vi "Handle Error SM.vi"(7 "NoContinue (F)":bool, 8 "error in (no error)":errorcluster, 10 "CustomMessage":string) -> (0 "error out":errorcluster, 1 "error out Upstream":errorcluster, 2 "Shutdown?":bool)   [LabVIEW 2019, in "ErrorHandler.lvclass"]
doc: "Developed by Kevin Thompson\nkevin@thompsonengineering.net\n\nCopyright 2018\nThompson Engineering, LLC"
uses:
  ErrorHandler.lvclass
  TypeDef/HandleErrorSM - AppData--clustesr.ctl
  <vilib>/Utility/error.llb/DialogType.ctl
  TypeDef/ErrorRemote EventData.ctl
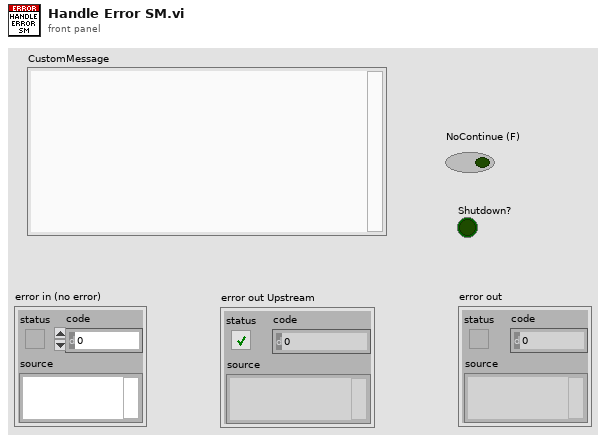
[diagram p1: front panel]
types:
  T1 = typedef "ErrorHandler.lvclass/HandleErrorSM - AppData--clustesr.ctl" = cluster{"error in":errorcluster, "ErrorText":string, "ErrorPathname":path, "ErrorRemoteEventData":T2}
  T2 = typedef "ErrorHandler.lvclass/ErrorRemote EventData.ctl" = cluster{"Timestamp":timestamp, "ErrorCluster":errorcluster, "message":string, "Shutdown?":bool, "DialogDisabled?":bool, "TerminateOnError?":bool}
  T3 = enum16{"Native", "Native Command Line", "UNIX", "Macintosh", "DOS"}
  T4 = typedef "DialogType.ctl" = u16
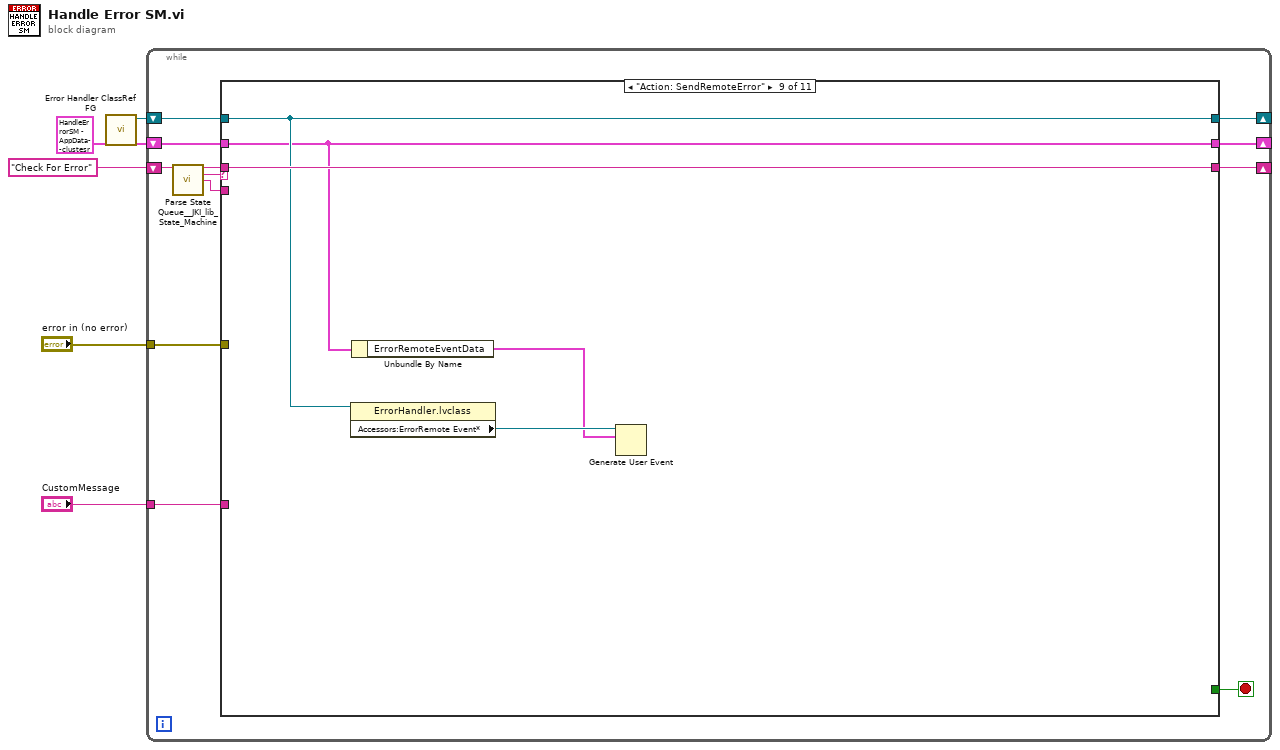
[diagram p0: block diagram]
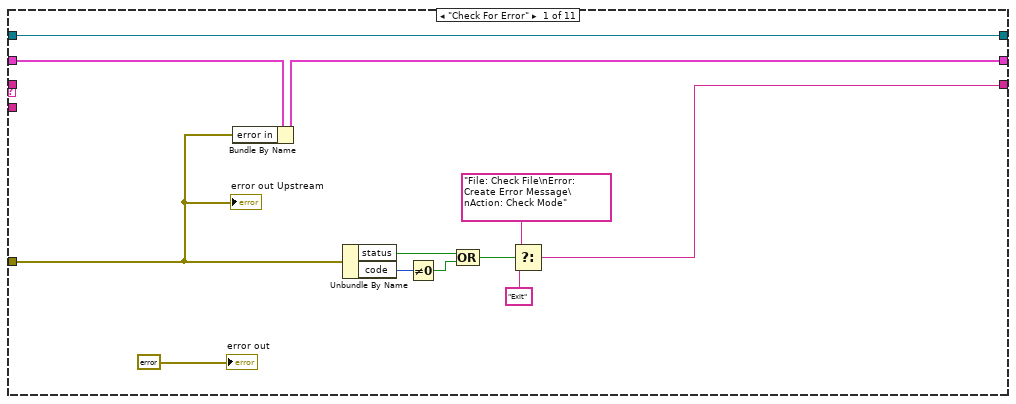
[diagram p2: hidden frame]
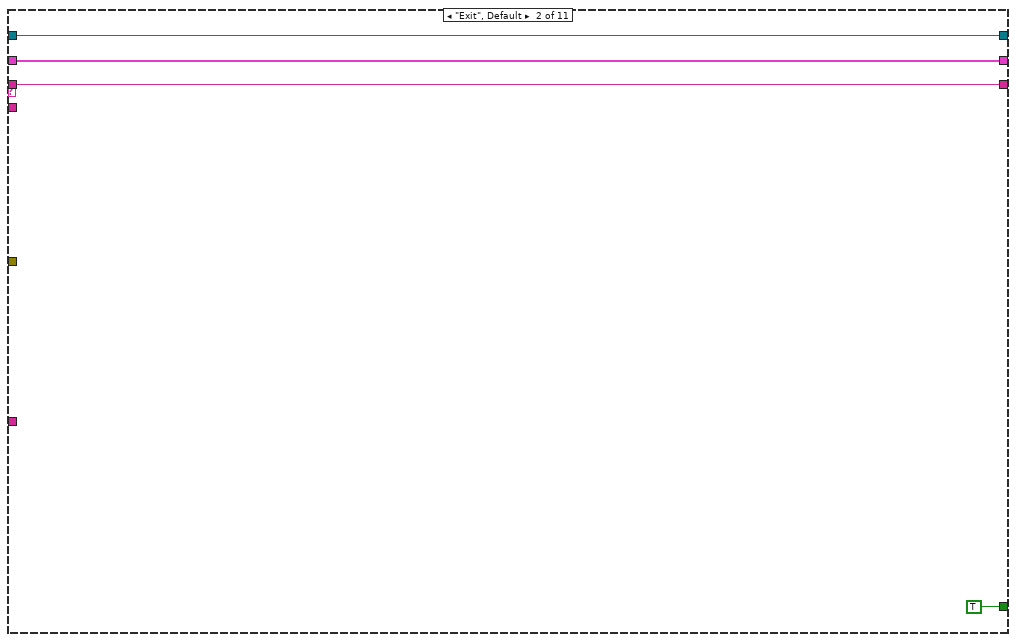
[diagram p3: hidden frame]
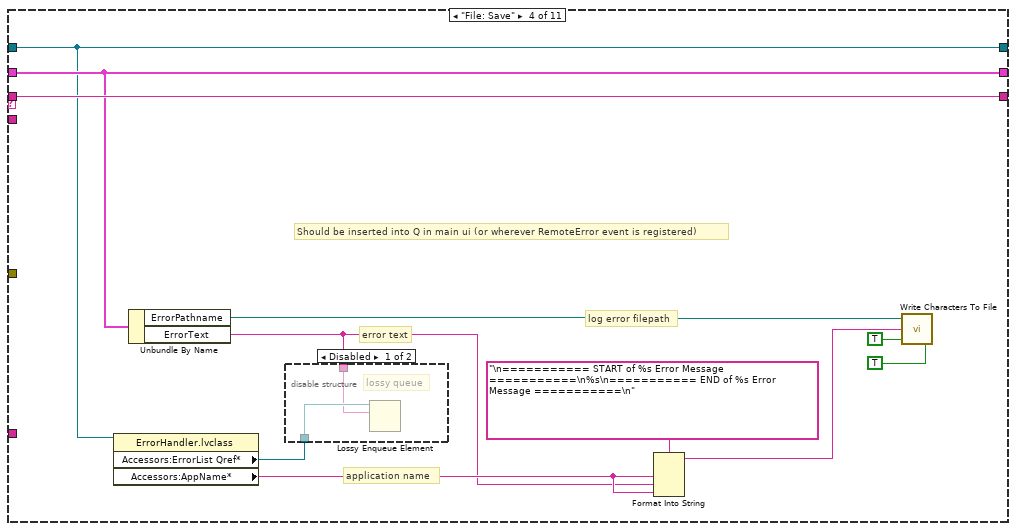
[diagram p5: hidden frame]
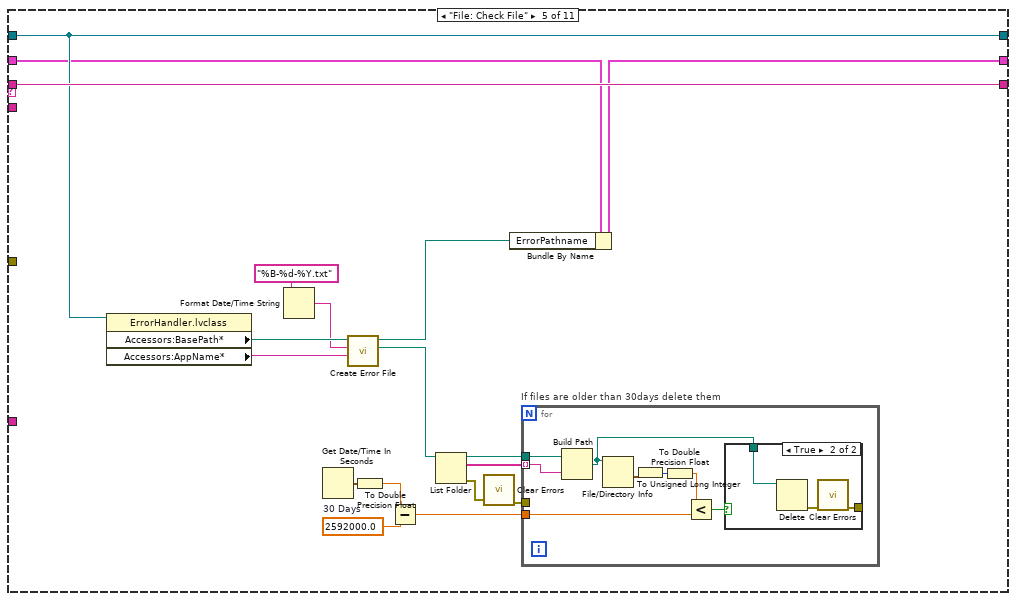
[diagram p7: hidden frame]
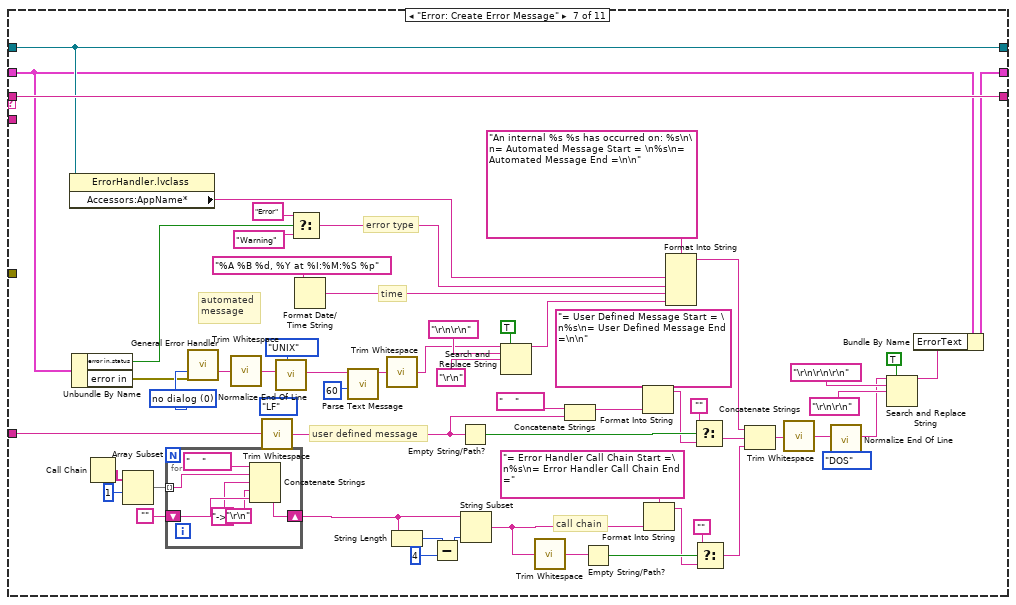
[diagram p10: hidden frame]
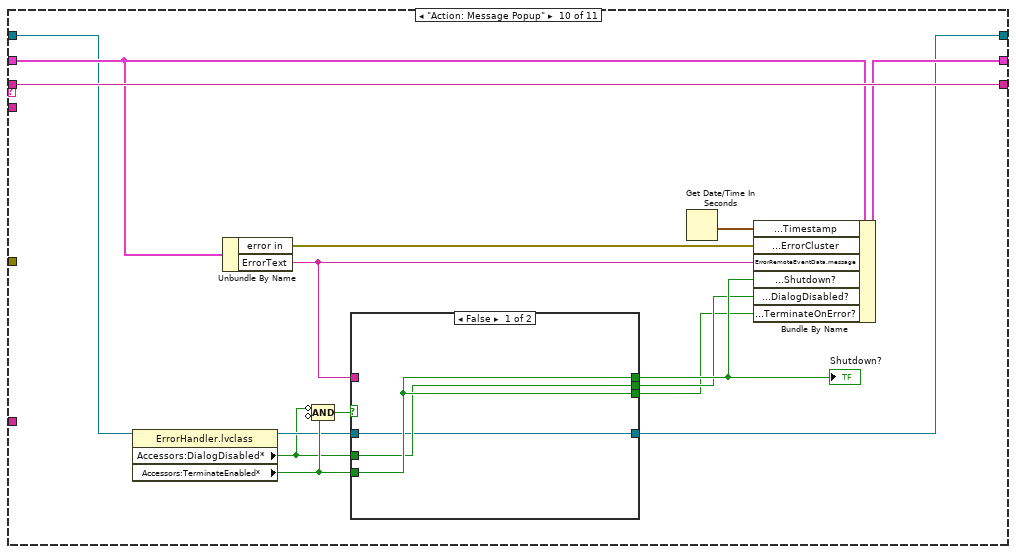
[diagram p12: hidden frame]
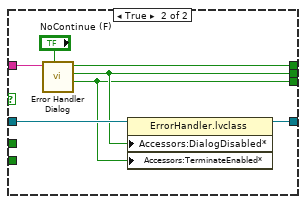
[diagram p13: hidden frame]
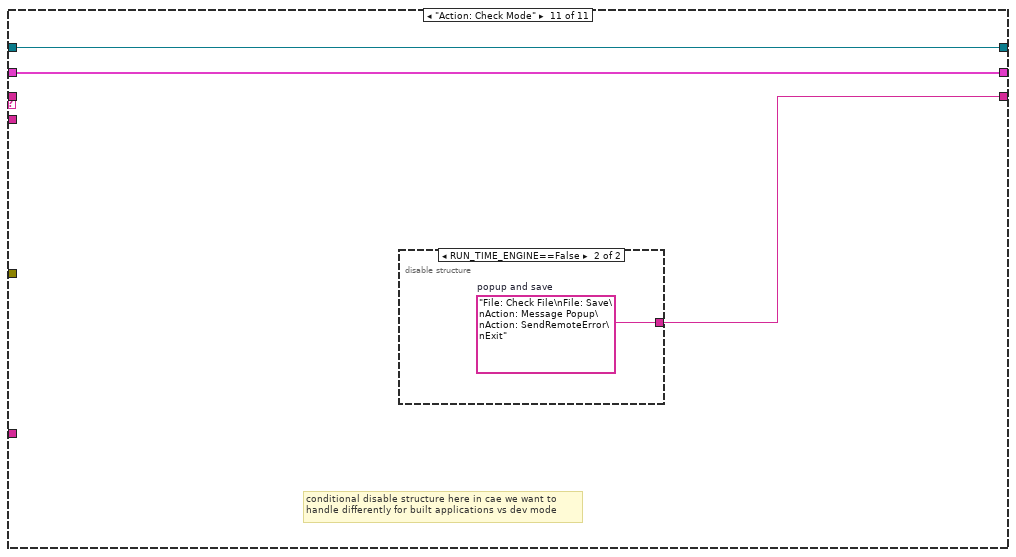
[diagram p14: hidden frame]
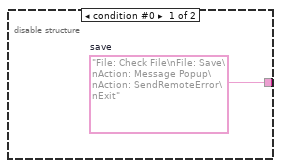
[diagram p15: hidden frame]
diagram:
  n1 = call "Error Handler ClassRef FG.vi"() -> ("ErrorHandler out"=w5:refnum<class "ErrorHandler.lvclass">)  [unwired: 10 in, 1 out]
  n2 = while {
    shift-right: [w14] -> _
    shift-left: "Check For Error" ("Remaining States") -> [w16]
    shift-right: [w11] -> _
    shift-left: w5 -> [w12]
    tunnel: "error in (no error)" -> [w10]
    shift-right: [w8] -> _
    shift-left: T1 {"error in"={"status"=FALSE, "code"=0, "source"=""}, "ErrorText"="", "ErrorPathname"=path "", "ErrorRemoteEventData"={"Timestamp"=timestamp(0 s since 1904-01-01), "ErrorCluster"={"status"=FALSE, "code"=0, "source"=""}, "message"="", "Shutdown?"=FALSE, "DialogDisabled?"=FALSE, "TerminateOnError?"=FALSE}} ("HandleErrorSM AppData") -> [w9]
    tunnel: "CustomMessage" -> [w6]
    stop <- w7 stop-if-true
    n3 = call <vilib>:"Parse State Queue__JKI_lib_State_Machine.vi"("State Queue"=w16) -> ("Remaining States"=w15:string, "Current State"=w17:string, "Arguments"=w13:string)  [unwired: 12 in]
    n4 = case shown="\"Action: SendRemoteError\"" w17 {
      tunnel: w15 -> [_ w33 w36 w47 w67 w81 w139 w148 w153 w168 _]
      tunnel: [w22 w33 w36 w47 w67 w81 w139 w148 w153 w168 w179] -> w14
      tunnel: w13 -> [_ _ _ _ _ _ _ _ _ _ _]
      tunnel: w12 -> [w29 w32 w35 w40 w66 w80 w91 w147 w152 w155 w181]
      tunnel: [w29 w32 w35 w40 w66 w80 w91 w147 w152 w154 w181] -> w11
      tunnel: w10 -> [w19 _ _ _ _ _ _ _ _ _ _]
      tunnel: [w20 w31 w34 w41 w51 w79 w87 w146 w150 w162 w180] -> w8
      tunnel: w9 -> [w21 w31 w34 w41 w52 w79 w88 w146 w150 w163 w180]
      tunnel: [_ TRUE _ _ _ _ _ _ _ _ _] -> w7
      tunnel: w6 -> [_ _ _ _ _ _ w89 _ _ _ _]
      frame "Check For Error" {
        n5 = Bundle By Name(cluster=w21, "error in"=w19) -> (w20:T1)
        n6 = Unbundle By Name(w19) -> ("status"=w28:bool, "code"=w27:i32)
        n7 = Not Equal To 0?(x=w27) -> (x != 0?=w26:bool)
        n8 = Compound Arithmetic op=OR(w28, w26) -> (w25:bool)
        n9 = Select(t="File: Check File\nError: Create Error Message\nAction: Check Mode", s=w25, f="Exit") -> (s? t:f=w22:string)
        "error out" <- errorcluster {"status"=FALSE, "code"=0, "source"=""} ("error constant")
        "error out Upstream" <- w19
      }
      frame "Exit", Default {
      }
      frame "------ File ------" {
      }
      frame "File: Save" {
        # "Should be inserted into Q in main ui (or wherever RemoteError event is registered)"
        # "log error filepath"
        # "error text"
        # "application name"
        n10 = property class="ErrorHandler.lvclass"(reference=w40) -> ("Accessors:ErrorList Qref*"=w38:refnum<queue>, "Accessors:AppName*"=w39:string)  [unwired: 1 in, 2 out]
        n11 = Unbundle By Name(w41) -> ("ErrorPathname"=w42:path, "ErrorText"=w37:string)
        n12 = disable-structure shown="Disabled" {
          disable-tunnel: w38 -> [w49 _]
          disable-tunnel: w37 -> [w48 _]
          frame Disabled {
            # "lossy queue"
            n13 = Lossy Enqueue Element(queue=w49, element=w48) -> ()  [unwired: 1 in, 4 out]
          }
          frame Enabled {
          }
        }
        n14 = Format Into String(format string="\n=========== START of %s Error Message ===========\n%s\n=========== END of %s Error Message ===========\n" ("string"), w39, w37, w39) -> (resulting string=w46:string)  [unwired: 2 in, 1 out]
        n15 = call <vilib>:"Write Characters To File.vi"("convert eol? (no:F)"=TRUE ("append to file? (new file:F)"), "append to file? (new file:F)"=TRUE, "character string"=w46, "file path (dialog if empty)"=w42) -> ()  [unwired: 1 in, 1 out]
      }
      frame "File: Check File" {
        w60 = 2592000.0  # 30 Days
        n16 = property class="ErrorHandler.lvclass"(reference=w66) -> ("Accessors:BasePath*"=w65:path, "Accessors:AppName*"=w64:string)  [unwired: 1 in, 2 out]
        n17 = Format Date/Time String(time format string (%c)="%B-%d-%Y.txt") -> (date/time string=w53:string)  [unwired: 2 in]
        n18 = Get Date/Time In Seconds() -> (seconds since 1Jan1904=w61:timestamp)
        n19 = call "Create Error File.vi"("App Name"=w64, "File Name"=w53, "base path for error folder"=w65) -> ("Error Folder"=w55:path, "Error Pathname"=w50:path)  [unwired: 7 in]
        n20 = To Double Precision Float(number=w61) -> (double precision float=w58:dbl)
        n21 = Subtract(x=w58, y=w60) -> (x-y=w59:dbl)
        n22 = List Folder(path=w55) -> (path out=w56:path, filenames=w57:string[], error out=w62:errorcluster)  [unwired: 3 in, 1 out]
        n23 = call <vilib>:"Clear Errors.vi"("error in (no error)"=w62) -> ("error out"=w63:errorcluster)  [unwired: 5 in, 1 out]
        n24 = Bundle By Name(cluster=w52, "ErrorPathname"=w50) -> (w51:T1)
        n25 = for "If files are older than 30days delete them" {
          tunnel: w56 -> [w75]
          tunnel: w57 -> [w74] mode=indexing
          tunnel: w59 -> [w72]
          tunnel: w63 -> [_]
          n26 = Build Path(base path=w75, name or relative path=w74) -> (appended path=w69:path)
          n27 = File/Directory Info(path=w69) -> (last mod=w68:timestamp)  [unwired: 1 in, 6 out]
          n28 = To Unsigned Long Integer(number=w68) -> (unsigned 32bit integer=w73:u32)
          n29 = To Double Precision Float(number=w73) -> (double precision float=w71:dbl)
          n30 = Less?(x=w71, y=w72) -> (x < y?=w70:bool)
          n31 = case shown="True" w70 {
            tunnel: w69 -> [_ w78]
            tunnel: [_ w76] -> _
            frame False {
            }
            frame True {
              n32 = Delete(path (use dialog)=w78) -> (error out=w77:errorcluster)  [unwired: 4 in, 2 out]
              n33 = call <vilib>:"Clear Errors.vi"("error in (no error)"=w77) -> ("error out"=w76:errorcluster)  [unwired: 5 in, 1 out]
            }
          }
        }
      }
      frame "------ Error ------" {
      }
      frame "Error: Create Error Message" {
        (unwired) enum16{"CR", "LF", "CRLF"}."LF" ("Convert to:")
        w133 = T4 0 items=["no dialog", "OK message", "continue or stop message", "OK message + warnings", "continue/stop + warnings"] ("type of dialog (OK msg:1)")
        # "call chain"
        # "automated\nmessage"
        # "user defined message"
        # "error type"
        # "time"
        n34 = property class="ErrorHandler.lvclass"(reference=w91) -> ("Accessors:AppName*"=w90:string)  [unwired: 1 in, 2 out]
        n35 = Unbundle By Name(w88) -> ("error in.status"=w132:bool, "error in"=w130:errorcluster)
        n36 = Call Chain() -> (call chain=w118:string[])
        n37 = Array Subset(array=w118, index=1 ("Array Index")) -> (w117:string[])  [unwired: 1 in]
        n38 = for {
          tunnel: w117 -> [w144] mode=indexing
          shift-right: [w142] -> w115
          shift-left: "" -> [w145]
          n39 = Concatenate Strings("    ", w144, "->" ("Substring"), "\r\n", w145) -> (w142:string)
        }
        n40 = call <vilib>:"General Error Handler.vi"("type of dialog (OK msg:1)"=w133, "error in (no error)"=w130) -> ("message"=w123:string)  [unwired: 9 in, 4 out]
        n41 = call <vilib>:"Trim Whitespace.vi"("string"=w123) -> ("trimmed string"=w95:string)  [unwired: 1 in]
        n42 = call <vilib>:"Trim Whitespace.vi"("string"=w89) -> ("trimmed string"=w114:string)  [unwired: 1 in]
        n43 = call <vilib>:"Normalize End Of Line.vi"("end of line (Native)"=T3."UNIX", "string in"=w95) -> ("string out"=w85:string)  [unwired: 6 in]
        n44 = Select(t="Error" ("Substring"), s=w132, f="Warning" ("Substring")) -> (s? t:f=w122:string)
        n45 = Format Date/Time String(time format string (%c)="%A %B %d, %Y at %I:%M:%S %p" ("Substring")) -> (date/time string=w128:string)  [unwired: 2 in]
        n46 = call "Parse Text Message.vi"("Characters Per Line"=60, "Input String"=w85) -> ("Output String"=w84:string)  [unwired: 8 in, 1 out]
        n47 = call <vilib>:"Trim Whitespace.vi"("string"=w84) -> ("trimmed string"=w98:string)  [unwired: 1 in]
        n48 = String Length(string=w115) -> (length=w136:i32)
        n49 = Subtract(x=w136, y=4) -> (x-y=w134:i32)
        n50 = Empty String/Path?(string/path=w114) -> (empty?=w126:bool)
        n51 = String Subset(string=w115, length (rest)=w134) -> (substring=w110:string)  [unwired: 1 in]
        n52 = Search and Replace String(replace all?=TRUE ("replace all? (F)"), input string=w98, search string="\r\n\r\n" ("String"), replace string="\r\n" ("String")) -> (result string=w97:string)  [unwired: 4 in, 3 out]
        n53 = call <vilib>:"Trim Whitespace.vi"("string"=w110) -> ("trimmed string"=w111:string)  [unwired: 1 in]
        n54 = Concatenate Strings("    ", w114) -> (w112:string)
        n55 = Empty String/Path?(string/path=w111) -> (empty?=w106:bool)
        n56 = Format Into String(format string="= User Defined Message Start = \n%s\n= User Defined Message End =\n\n", w112) -> (resulting string=w125:string)  [unwired: 2 in, 1 out]
        n57 = Format Into String(format string="= Error Handler Call Chain Start =\n%s\n= Error Handler Call Chain End =", w110) -> (resulting string=w82:string)  [unwired: 2 in, 1 out]
        n58 = Format Into String(format string="An internal %s %s has occurred on: %s\n\n= Automated Message Start = \n%s\n= Automated Message End =\n\n", w90, w122, w128, w97) -> (resulting string=w105:string)  [unwired: 2 in, 1 out]
        n59 = Select(t="", s=w126, f=w125) -> (s? t:f=w104:string)
        n60 = Select(t="", s=w106, f=w82) -> (s? t:f=w103:string)
        n61 = Concatenate Strings(w105, w104, w103) -> (w102:string)
        n62 = call <vilib>:"Trim Whitespace.vi"("string"=w102) -> ("trimmed string"=w92:string)  [unwired: 1 in]
        n63 = call <vilib>:"Normalize End Of Line.vi"("end of line (Native)"=T3."DOS", "string in"=w92) -> ("string out"=w93:string)  [unwired: 6 in]
        n64 = Search and Replace String(replace all?=TRUE ("replace all? (F)"), input string=w93, search string="\r\n\r\n\r\n" ("String"), replace string="\r\n\r\n" ("String")) -> (result string=w86:string)  [unwired: 4 in, 3 out]
        n65 = Bundle By Name(cluster=w88, "ErrorText"=w86) -> (w87:T1)
      }
      frame "------ Action ------" {
      }
      frame "Action: SendRemoteError" {
        n66 = property class="ErrorHandler.lvclass"(reference=w152) -> ("Accessors:ErrorRemote Event*"=w151:refnum<user-event>)  [unwired: 1 in, 2 out]
        n67 = Unbundle By Name(w150) -> ("ErrorRemoteEventData"=w149:T2)
        n68 = Generate User Event(user event=w151, event data cluster=w149) -> ()  [unwired: 2 in, 2 out]
      }
      frame "Action: Message Popup" {
        n69 = property class="ErrorHandler.lvclass"(reference=w155) -> (reference out=w165:refnum<class "ErrorHandler.lvclass">, "Accessors:DialogDisabled*"=w164:bool, "Accessors:TerminateEnabled*"=w166:bool)  [unwired: 1 in, 1 out]
        n70 = Unbundle By Name(w163) -> ("error in"=w158:errorcluster, "ErrorText"=w160:string)
        n71 = Compound Arithmetic op=AND(invert w164, invert w166) -> (w167:bool)
        n72 = case shown="False" w167 {
          tunnel: w166 -> [w171 _]
          tunnel: [w171 w177] -> w159
          tunnel: w160 -> [_ w178]
          tunnel: w165 -> [w169 w176]
          tunnel: [w170 w175] -> w157
          tunnel: [w171 w174] -> w156
          tunnel: w164 -> [w170 _]
          tunnel: [w169 w172] -> w154
          frame False {
          }
          frame True {
            n73 = call "Error Handler Dialog.vi"("NoContinue (F)"="NoContinue (F)", "ErrorText"=w178) -> ("TerminateApp?"=w174:bool, "DisableDialog?"=w175:bool, "Shutdown?"=w177:bool)  [unwired: 7 in]
            n74 = property class="ErrorHandler.lvclass"(reference=w176, "Accessors:DialogDisabled*"=w175, "Accessors:TerminateEnabled*"=w174) -> (reference out=w172:refnum<class "ErrorHandler.lvclass">)  [unwired: 1 in, 1 out]
          }
        }
        "Shutdown?" <- w159
        n75 = Get Date/Time In Seconds() -> (seconds since 1Jan1904=w161:timestamp)
        n76 = Bundle By Name(cluster=w163, "ErrorRemoteEventData.Timestamp"=w161, "ErrorRemoteEventData.ErrorCluster"=w158, "ErrorRemoteEventData.message"=w160, "ErrorRemoteEventData.Shutdown?"=w159, "ErrorRemoteEventData.DialogDisabled?"=w157, "ErrorRemoteEventData.TerminateOnError?"=w156) -> (w162:T1)
      }
      frame "Action: Check Mode" {
        # "conditional disable structure here in cae we want to\nhandle differently for built applications vs dev mode"
        n77 = disable-structure shown="RUN_TIME_ENGINE==False" {
          disable-tunnel: [w182 w183] -> w179
          frame condition #0 {
            w182 = "File: Check File\nFile: Save\nAction: Message Popup\nAction: SendRemoteError\nExit"  # save
          }
          frame condition #1 (active) {
            w183 = "File: Check File\nFile: Save\nAction: Message Popup\nAction: SendRemoteError\nExit"  # popup and save
          }
        }
      }
    }
  }
